vi "Replace.vi"(8 "error in (no error)":errorcluster, 11 "CConfig Nonpersistant Buffer in":refnum<class "CConfig Nonpersistant Buffer.lvclass">) -> (0 "error out":errorcluster, 2 "Replace?":bool=TRUE, 3 "CConfig Nonpersistant Buffer out":refnum<class "CConfig Nonpersistant Buffer.lvclass">)   [LabVIEW 2013, in "CConfig Nonpersistant Buffer.lvclass"]
doc: "Copyright 2018, Carya Automatisering, Wiebe Walstra."
uses:
  CConfig Nonpersistant Buffer.lvclass
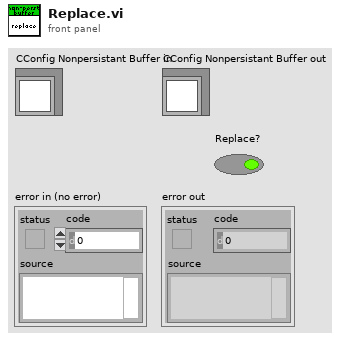
[diagram p1: front panel]
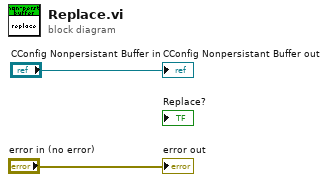
[diagram p0: block diagram]
diagram:
  "error out" <- "error in (no error)"
  "CConfig Nonpersistant Buffer out" <- "CConfig Nonpersistant Buffer in"
